vi "SaveAs.vi"(8 "error in":errorcluster, 11 "state in":T1) -> (0 "error out":errorcluster, 1 "canceled?":bool, 3 "state out":T1)   [LabVIEW 2019, in "Configuration Tool.lvlib"]
doc: "Calls the Save Dialog VI, and if a valid names is given calls the save function."
uses:
  Configuration Tool.lvlib
  Controls/StateCluster.ctl
  <vilib>/NI/Configuration Framework/Repository/NISE_CEF_Repository.lvclass
  <vilib>/NI/Configuration Framework/Node/NodeRef.ctl
  <vilib>/NI/Configuration Framework/Node/NISE_CEF_Node.lvclass
  <vilib>/NI/Configuration Framework/Node/StandardEvents.ctl
  <vilib>/NI/Configuration Framework/Node/UserEventRef.ctl
  <vilib>/NI/Configuration Framework/Controls/EventCluster.ctl
  <vilib>/NI/Configuration Framework/Node/NodeChangeEvent.ctl
  <vilib>/NI/Configuration Framework/Node/CacheState.ctl
  <vilib>/NI/Configuration Framework/Node/RefreshUIEvent.ctl
  <vilib>/NI/Configuration Framework/Node/StopEvent.ctl
  <vilib>/NI/Configuration Framework/glyph manager/glyph manager.ctl
  <vilib>/picture/picture.llb/imagedata.ctl
  <vilib>/NI/Configuration Framework/NISE_CEF_TreeControl.lvlib
  <vilib>/NI/Configuration Framework/glyph manager/glyph manager.lvlib
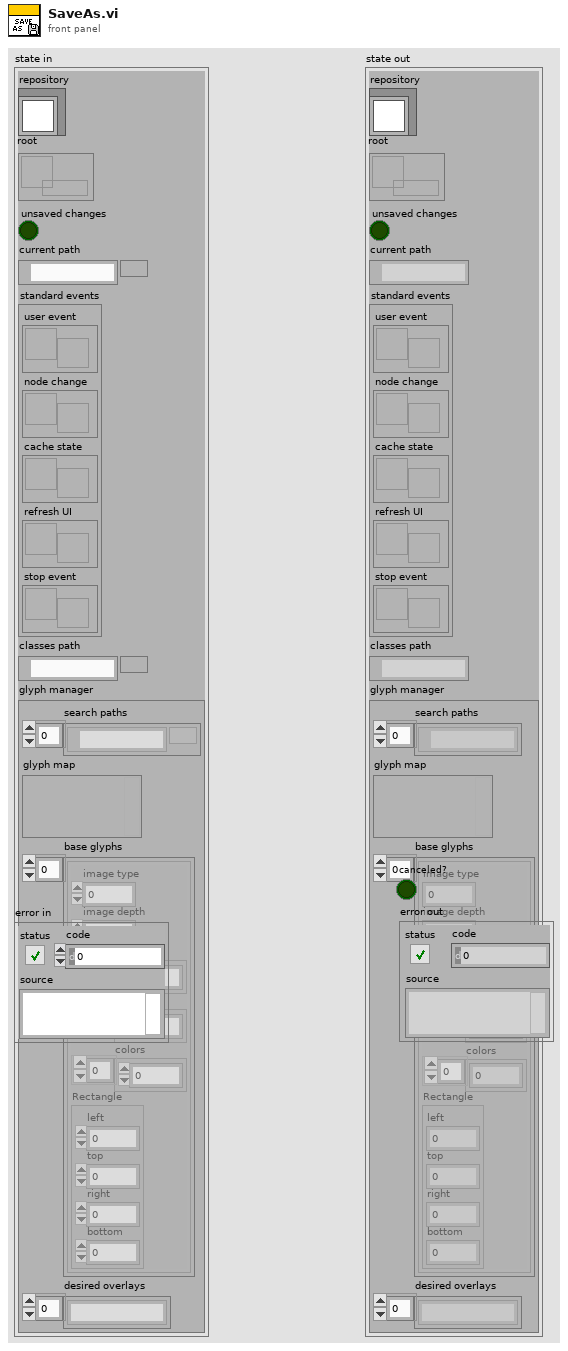
[diagram p1: front panel]
types:
  T1 = typedef "Configuration Tool.lvlib/StateCluster.ctl" = cluster{"repository":refnum<class "NISE_CEF_Repository.lvclass">, "root":T2, "unsaved changes":bool, "current path":path, "standard events":T3, "classes path":path, "glyph manager":T9}
  T2 = typedef "NISE_CEF_Node.lvclass/NodeRef.ctl" = refnum<data-value>
  T3 = typedef "NISE_CEF_Node.lvclass/StandardEvents.ctl" = cluster{"user event":T4, "node change":T5, "cache state":T6, "refresh UI":T7, "stop event":T8}
  T4 = typedef "NISE_CEF_Node.lvclass/UserEventRef.ctl" = refnum<user-event>
  T5 = typedef "NISE_CEF_Node.lvclass/NodeChangeEvent.ctl" = refnum<user-event>
  T6 = typedef "NISE_CEF_Node.lvclass/CacheState.ctl" = refnum<user-event>
  T7 = typedef "NISE_CEF_Node.lvclass/RefreshUIEvent.ctl" = refnum<user-event>
  T8 = typedef "NISE_CEF_Node.lvclass/StopEvent.ctl" = refnum<user-event>
  T9 = typedef "glyph manager.lvlib/glyph manager.ctl" = cluster{"search paths":path[], "glyph map":variant, "base glyphs":T10[], "desired overlays":string[]}
  T10 = typedef "imagedata.ctl" = cluster{"image type":i32, "image depth":i32, "image":u8[], "mask":u8[], "colors":u32[], "Rectangle":cluster{"left":i16, "top":i16, "right":i16, "bottom":i16}}
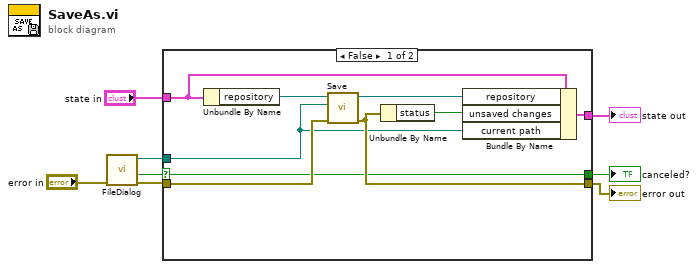
[diagram p0: block diagram]
diagram:
  n1 = call "FileDialog.vi"("error in"="error in") -> ("error out"=w4:errorcluster, "cancelled"=w2:bool, "selected path"=w3:path)  [unwired: 8 in]
  n2 = case shown="False" w2 {
    selector: w2 -> [w9 w19]
    tunnel: "state in" -> [w14 w20]
    tunnel: w4 -> [w13 w18]
    tunnel: [w12 w18] -> w7
    tunnel: [w11 w20] -> w6
    tunnel: w3 -> [w10 _]
    tunnel: [w9 w19] -> w1
    frame False {
      n3 = Unbundle By Name(w14) -> ("repository"=w17:refnum<class "NISE_CEF_Repository.lvclass">)
      n4 = call-dynamic "Save.vi"("error in"=w13, "file path"=w10, "repository in"=w17) -> ("error out"=w12:errorcluster, "repository out"=w15:refnum<class "NISE_CEF_Repository.lvclass">)  [unwired: 7 in]
      n5 = Unbundle By Name(w12) -> ("status"=w16:bool)
      n6 = Bundle By Name(cluster=w14, "repository"=w15, "unsaved changes"=w16, "current path"=w10) -> (w11:T1)
    }
    frame True {
    }
  }
  "state out" <- w6
  "error out" <- w7
  "canceled?" <- w1
